vi "Calculate Forces.vi"(7 "Integrator Reset":bool, 8 "error in (no error)":errorcluster, 10 "Vessel in":refnum<class "Vessel.lvclass">, 11 "Oculus Rift Controller in":refnum<class "Oculus Rift Controller.lvclass">) -> (0 "error out":errorcluster, 2 "Vessel out":refnum<class "Vessel.lvclass">, 3 "Oculus Rift Controller out":refnum<class "Oculus Rift Controller.lvclass">)   [LabVIEW 2014, in "Controller Library.lvlib" / "Oculus Rift Controller.lvclass"]
doc: "This VI calculates the forces in each controlled degree of freedom direction to follow a desired path or point."
uses:
  Oculus Rift Controller.lvclass
  ROV/Vessel.lvclass
  Supervisor/Supervisor.lvclass
panel:
  in  "SET MANUAL control":bool
  in  "SET MANUAL depth":bool
  in  "delta HEAD REF":dbl
  in  "delta  DEPTH REF":dbl
  in  "PID gains depth":T1={"proportional gain (Kc)"=500.0, "integral time (Ti, min)"=0.83, "derivative time (Td, min)"=0.01} {"derivative time (Td, min)" format="%.3f"; "integral time (Ti, min)" format="%.3f"; "proportional gain (Kc)" format="%.3f"}
  in  "Auto Depth":bool
  in  "Auto Heading":bool
  in  "PID gains head":T1={"proportional gain (Kc)"=150.0, "integral time (Ti, min)"=0.5, "derivative time (Td, min)"=0.008} {"derivative time (Td, min)" format="%.3f"; "integral time (Ti, min)" format="%.3f"; "proportional gain (Kc)" format="%.3f"}
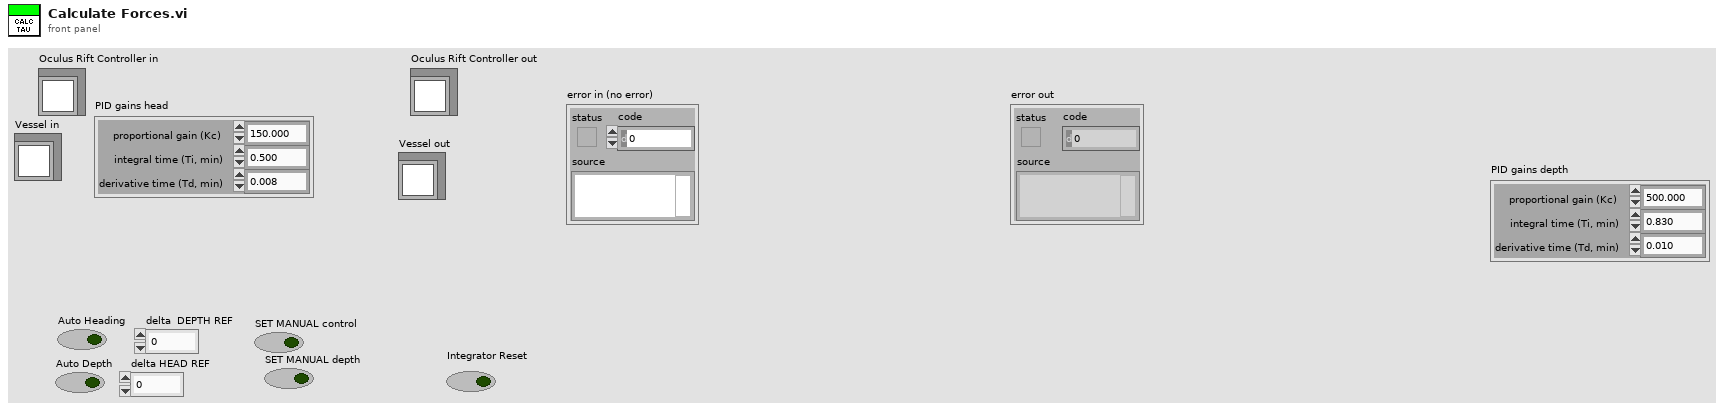
[diagram p1: front panel]
types:
  T1 = cluster{"proportional gain (Kc)":dbl, "integral time (Ti, min)":dbl, "derivative time (Td, min)":dbl}
  T2 = cluster{"Measured":cluster{"Eta":dbl[], "Nu":dbl[], "Eta Dot":dbl[], "Nu Dot":dbl[]}, "Estimated":cluster{"Eta":dbl[], "Nu":dbl[], "Eta Dot":dbl[], "Nu Dot":dbl[]}, "Desired":cluster{"Eta":dbl[], "Nu":dbl[], "Eta Dot":dbl[], "Nu Dot":dbl[]}, "Previous Desired":cluster{"Eta":dbl[], "Nu":dbl[], "Eta Dot":dbl[], "Nu Dot":dbl[]}, "tau":dbl[], "Altitude":cluster{"Measured":dbl, "Estimated":dbl, "Desired":dbl, "Previous Desired":dbl, "Approximated":dbl, "grad F":dbl[]}, "rpm":dbl[], "Attitude":cluster{"Theta Measured":dbl[], "Theta Estimated":dbl[], "Omega Measured":dbl[], "Omega Estimated":dbl[], "Gyro Bias":dbl[]}}
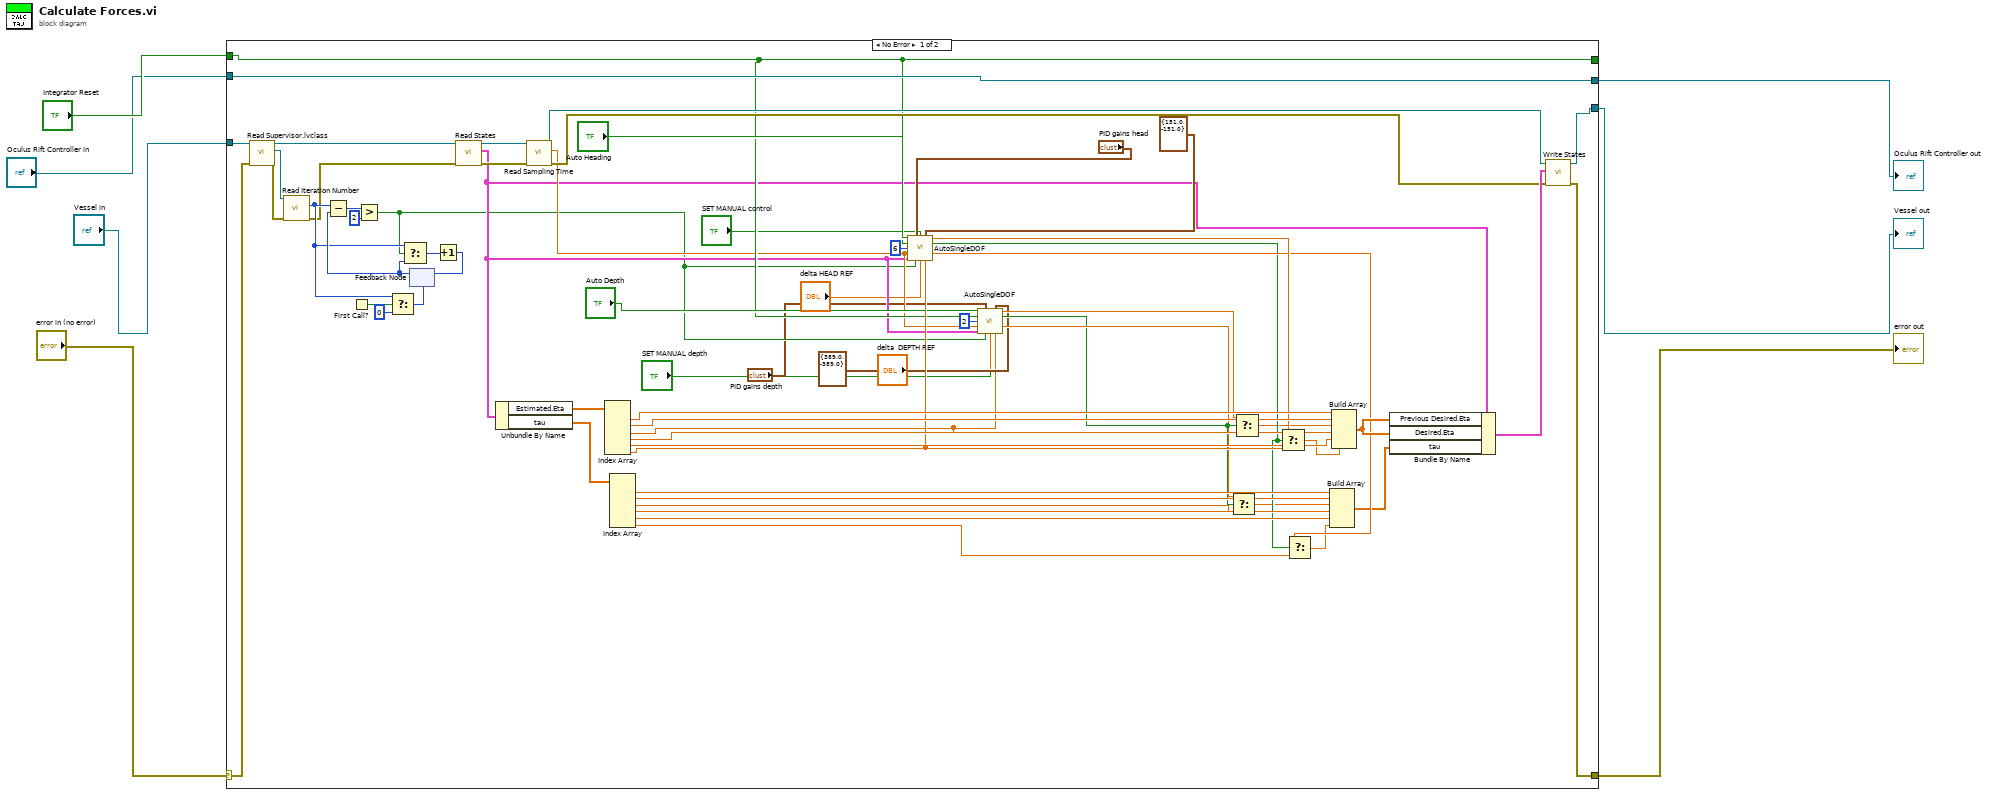
[diagram p0: block diagram]
diagram:
  n1 = case shown="No Error" "error in (no error)" {
    selector: "error in (no error)" -> [w34 w76]
    tunnel: [w29 w76] -> w5
    tunnel: [w27 w75] -> _
    tunnel: "Integrator Reset" -> [w27 w75]
    tunnel: "Vessel in" -> [w37 w74]
    tunnel: [w67 w74] -> w6
    tunnel: [w72 w73] -> w2
    tunnel: "Oculus Rift Controller in" -> [w72 w73]
    frame No Error {
      n2 = call "Read Supervisor.lvclass.vi"("error in (no error)"=w34, "Vessel in"=w37) -> ("error out"=w33:errorcluster, "Supervisor.lvclass"=w35:refnum<class "Supervisor.lvclass">, "Vessel out"=w36:refnum<class "Vessel.lvclass">)  [unwired: 7 in]
      n3 = call-dynamic "Read Iteration Number.vi"("error in (no error)"=w33, "Supervisor in"=w35) -> ("error out"=w32:errorcluster, "Iteration Number"=w39:i32)  [unwired: 7 in, 1 out]
      n4 = First Call?() -> (First Call?: T/F=w45:bool)
      n5 = Select(t=w39, s=w45, f=0) -> (s? t:f=w43:i32)
      n6 = feedback #1(w43) -> (w40:i32)
      n7 = Subtract(x=w39, y=w40) -> (x-y=w46:i32)
      n8 = Greater?(x=w46, y=2) -> (0:w17:bool)
      n9 = Select(t=w39, s=w17, f=w40) -> (s? t:f=w42:i32)
      n10 = Increment(x=w42) -> (x+1=w41:i32)
      n11 = feedback-in #1(w41) -> ()
      n12 = call-dynamic "Read States.vi"("error in (no error)"=w32, "Vessel in"=w36) -> ("error out"=w31:errorcluster, "States"=w25:T2, "Vessel out"=w65:refnum<class "Vessel.lvclass">)  [unwired: 7 in]
      n13 = Unbundle By Name(w25) -> ("Estimated.Eta"=w70:dbl[], "tau"=w56:dbl[])
      n14 = call-dynamic "Read Sampling Time.vi"("error in (no error)"=w31, "Vessel in"=w65) -> ("error out"=w30:errorcluster, "Sampling Time"=w26:dbl, "Vessel out"=w68:refnum<class "Vessel.lvclass">)  [unwired: 7 in]
      n15 = Index Array(array=w70) -> (element #1=w64:dbl, element #2=w63:dbl, element #3=w12:dbl, element #4=w62:dbl, element #5=w60:dbl, element #6=w57:dbl)  [unwired: 6 in]
      n16 = Index Array(array=w56) -> (element #1=w55:dbl, element #2=w54:dbl, element #3=w24:dbl, element #4=w51:dbl, element #5=w53:dbl, element #6=w18:dbl)  [unwired: 6 in]
      n17 = call "AutoSingleDOF.vi"("Auto Heading"="Auto Heading", "PID gains head"="PID gains head", "SET MANUAL"="SET MANUAL control", "output range"=cluster{"output high":dbl, "output low":dbl} {"output high"=151.0, "output low"=-151.0}, "Integrator Reset"=w27, "varNumber"=6, "Sampling Time"=w26, "States"=w25, "Boolean"=w17, "delta REF"="delta HEAD REF", "Numeric"=w57) -> ("set point"=w58:dbl, "auto set"=w38:bool, "output"=w52:dbl)  [unwired: 2 in]
      n18 = call "AutoSingleDOF.vi"("Auto Heading"="Auto Depth", "PID gains head"="PID gains depth", "SET MANUAL"="SET MANUAL depth", "output range"=cluster{"output high":dbl, "output low":dbl} {"output high"=389.0, "output low"=-389.0}, "Integrator Reset"=w27, "varNumber"=2, "Sampling Time"=w26, "States"=w25, "Boolean"=w17, "delta REF"="delta  DEPTH REF", "Numeric"=w12) -> ("set point"=w21:dbl, "auto set"=w20:bool, "output"=w22:dbl)  [unwired: 2 in]
      n19 = Select(t=w22, s=w20, f=w24) -> (s? t:f=w23:dbl)
      n20 = Select(t=w21, s=w20, f=w12) -> (s? t:f=w19:dbl)
      n21 = Select(t=w58, s=w38, f=w57) -> (s? t:f=w59:dbl)
      n22 = Select(t=w52, s=w38, f=w18) -> (s? t:f=w50:dbl)
      n23 = Build Array(w55, w54, w23, w51, w53, w50) -> (w49:dbl[])
      n24 = Build Array(w64, w63, w19, w62, w60, w59) -> (w61:dbl[])
      n25 = Bundle By Name(cluster=w25, "Previous Desired.Eta"=w61, "Desired.Eta"=w61, "tau"=w49) -> (w66:T2)
      n26 = call-dynamic "Write States.vi"("error in (no error)"=w30, "States"=w66, "Vessel in"=w68) -> ("error out"=w29:errorcluster, "Vessel out"=w67:refnum<class "Vessel.lvclass">)  [unwired: 7 in]
    }
    frame Error {
    }
  }
  "error out" <- w5
  "Oculus Rift Controller out" <- w2
  "Vessel out" <- w6
